vi "v5.41.vi"() -> ()   [LabVIEW 2018]
uses:
  <vilib>/DAQmx/read.llb/DAQmx Read (Analog 1D DBL NChan 1Samp).vi
  <extravilib>/ChannelInstances/Lossy Stream-c(a[.](c(dbl,dbl,dbl,dbl)),stamp,a[.](dbl),c(dbl,dbl,dbl,dbl,dbl,dbl,dbl))/Read With Abort.vi
  <extravilib>/ChannelInstances/High Speed Stream-c(a[.](c(dbl,dbl,dbl,dbl)),stamp,a[.](dbl),c(dbl,dbl,dbl,dbl,dbl,dbl,dbl))/_Read For Replicate.vi
  <extravilib>/ChannelInstances/Lossy Stream-c(a[.](c(dbl,dbl,dbl,dbl)),stamp,a[.](dbl),c(dbl,dbl,dbl,dbl,dbl,dbl,dbl))/Write With Abort.vi
  <extravilib>/ChannelInstances/Lossy Stream-c(a[.](c(dbl,dbl,dbl,dbl)),stamp,a[.](dbl),c(dbl,dbl,dbl,dbl,dbl,dbl,dbl))/EndpointRead.vi
  <extravilib>/ChannelInstances/Lossy Stream-c(a[.](c(dbl,dbl,dbl,dbl)),stamp,a[.](dbl),c(dbl,dbl,dbl,dbl,dbl,dbl,dbl))/Endpoint.vi
  <extravilib>/ChannelInstances/Lossy Stream-c(a[.](c(dbl,dbl,dbl,dbl)),stamp,a[.](dbl),c(dbl,dbl,dbl,dbl,dbl,dbl,dbl))/Instantiate.vi
  <extravilib>/ChannelInstances/Lossy Stream-c(a[.](c(dbl,dbl,dbl,dbl)),stamp,a[.](dbl),c(dbl,dbl,dbl,dbl,dbl,dbl,dbl))/)Channel.vi
  <resource>/ChannelSupport/_ChannelSupport/WaitIfNeeded.vi
  <extravilib>/ChannelInstances/High Speed Stream-c(a[.](c(dbl,dbl,dbl,dbl)),stamp,a[.](dbl),c(dbl,dbl,dbl,dbl,dbl,dbl,dbl))/Instantiate.vi
  <extravilib>/ChannelInstances/High Speed Stream-c(a[.](c(dbl,dbl,dbl,dbl)),stamp,a[.](dbl),c(dbl,dbl,dbl,dbl,dbl,dbl,dbl))/)Channel.vi
  <extravilib>/ChannelInstances/High Speed Stream-c(a[.](c(dbl,dbl,dbl,dbl)),stamp,a[.](dbl),c(dbl,dbl,dbl,dbl,dbl,dbl,dbl))/Abort Signal/Init Signal.vi
  <vilib>/Utility/file.llb/Write Delimited Spreadsheet (string).vi
  <vilib>/DAQmx/create/channels.llb/DAQmx Create Channel (AI-Temperature-Thermocouple).vi
  <vilib>/DAQmx/configure/timing.llb/DAQmx Timing (Sample Clock).vi
  <vilib>/DAQmx/miscellaneous.llb/DAQmx Fill In Error Info.vi
  <extravilib>/ChannelInstances/High Speed Stream-c(a[.](c(dbl,dbl,dbl,dbl)),stamp,a[.](dbl),c(dbl,dbl,dbl,dbl,dbl,dbl,dbl)).lvlib
  <resource>/objmgr/daqmx.rc
  <extravilib>/ChannelInstances/Lossy Stream-c(a[.](c(dbl,dbl,dbl,dbl)),stamp,a[.](dbl),c(dbl,dbl,dbl,dbl,dbl,dbl,dbl)).lvlib
panel:
  in  "Rig Temperature Tab Box":enum32{"Rig Temps Live", "Alarm Thresholds"}(tab)
  out "Rig Temperatures":T1
  in  "Rig Alarm Thresholds":T1
  out "DAQ Current Time":timestamp format="%<%X>T"
  in  "UI Refresh Rate (Hz)":u32=1 min=1 max=500 step=1
  out "Line Pressures":T2(graph)
  in  "Boondoggle":dbl(slide) scale=0.0..10.0
  out "Line Temperatures":T2(graph)
  out "Stoichiometric AFR [g/s]":dbl
  in  "stop":bool
  in  "Species List":string[][](table)=[["Custom", "9999999999"], ["Methanol", "6.47"], ["Butanol", "11.2"], ["Diesel", "14.5"], ["Gasoline", "14.7"], ["Propane", "15.67"], ["Methane", "13.19"], ["Hydrogen", "34.3"], ["Ammonia", "6.0466"], ["Pentane", "15.32"], ["Butane", "14.98"], ["Hexane", "15.24"], ["Ethanol", "9"], ["Empty (Not Used)", "0"]]
  in  "Lines Tab Control\n(Don't delete)":enum32{"Live Data", "AFR Info", "Setup Lines"}(tab)
  out "Flowrate Data":T3(array[cluster])
  out "AFR Display":T4(array[cluster])
  in  "Line Setup":T5(array[cluster])
  out "Actual Sample Rate":dbl
  out "Export Timestamp":timestamp format="%<%H:%M:%S>T"
  out "UI Timestamp":timestamp format="%<%X\n%x>T"
  in  "file path (dialog if empty)":path
  out "Export Loop Status":T6(ring)
  in  "Start Recording?":bool
  in  "Stop Recording?":bool
  out "Aquisition\nLoop Status":T7(ring)
  in  "OK Button":bool
  in  "DAQ Properties":cluster{"Sample Rate [Hz]":dbl}={"Sample Rate [Hz]"=1.0} {"Sample Rate [Hz]" min=1.0 max=500.0 step=1.0}
  # "Rig Temperatures [ °C]"
  # "Rig Alarm Thresholds [ °C]"
  # "Live \n Live Line Data"
  # "Air-to-Fuel Ratios for each Line"
  # "Line Setup"
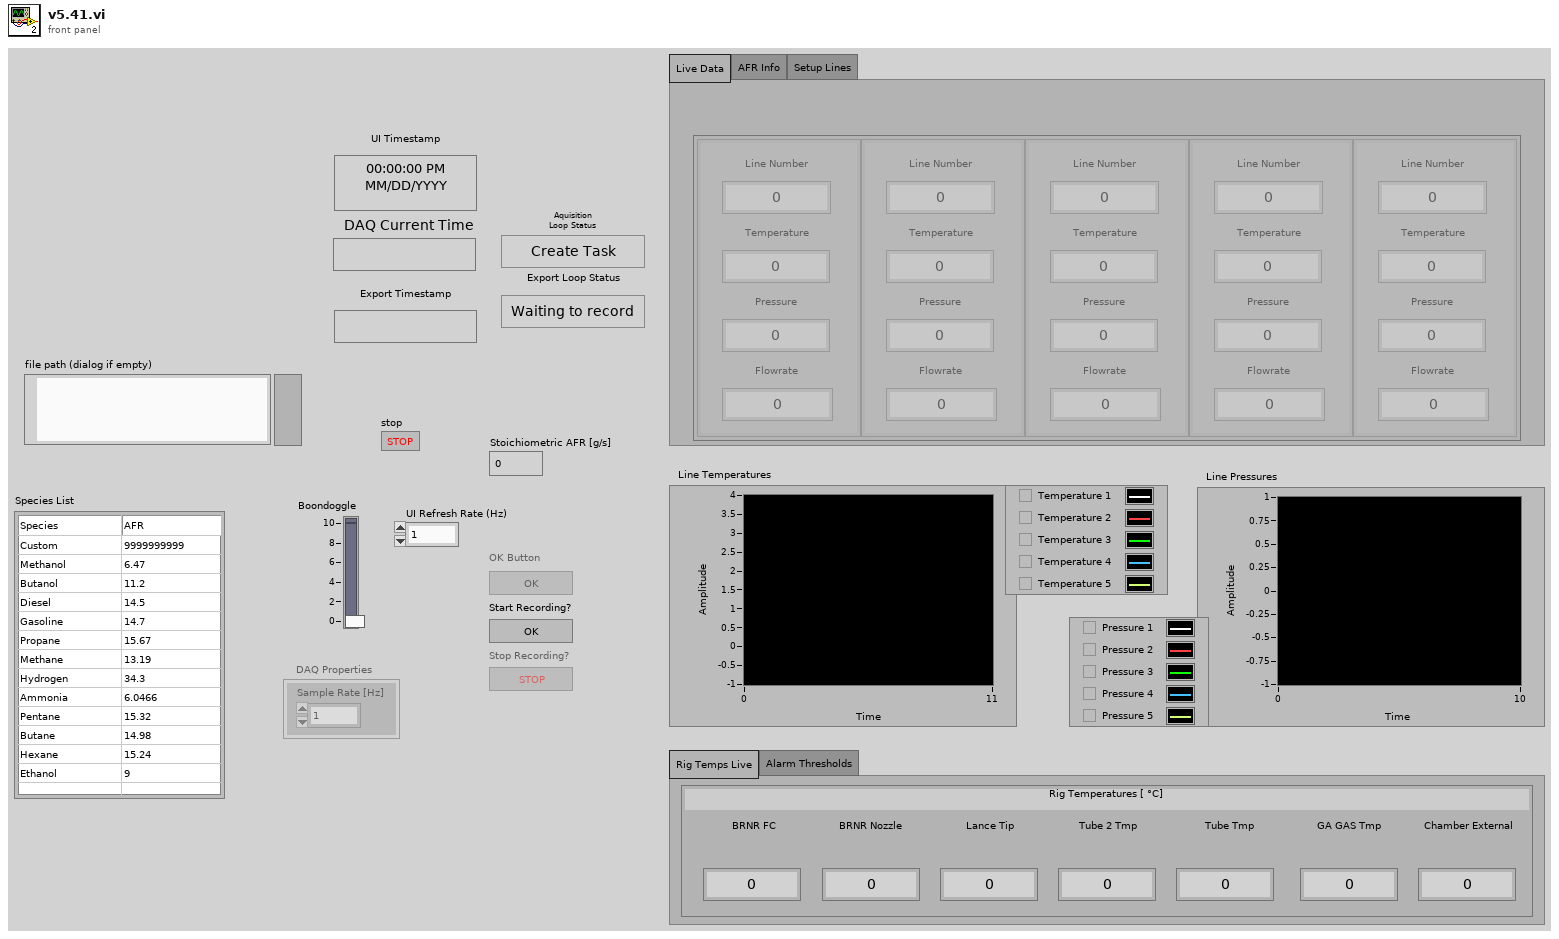
[diagram p1: front panel]
types:
  T1 = cluster{"BRNR FC":dbl, "BRNR Nozzle":dbl, "Lance Tip":dbl, "Tube 2 Tmp":dbl, "Tube Tmp":dbl, "GA GAS Tmp":dbl, "Chamber External":dbl}
  T2 = cluster{"[0]":dbl, "[1]":dbl, "[2]":dbl, "[3]":dbl, "[4]":dbl}
  T3 = cluster{"Line Number":dbl, "Temperature":dbl, "Pressure":dbl, "Flowrate":dbl}[]
  T4 = cluster{"Line Number":i32, "AFR":dbl, "Species":enum16{"Empty (Not used)", "Custom", "Methanol", "Ethanol", "Butanol", "Diesel", "Gasoline", "Propane", "Methane", "Hydrogen", "Pentane", "Butane", "Hexane"}}[]
  T5 = cluster{"Custom AFR":dbl, "Species":enum16{"Empty (Not used)", "Custom", "Methanol", "Ethanol", "Butanol", "Diesel", "Gasoline", "Propane", "Methane", "Hydrogen", "Pentane", "Butane", "Hexane"}}[]
  T6 = enum16{"Waiting to record", "Creating Spreadsheet", "Recording", "Finished Recording"}
  T7 = enum16{"Create Task", "Change Settings", "Check Settings", "Read Data", "End Task"}
  T8 = enum8{"Enabled", "Disabled", "Disabled and Grayed Out"}
  T9 = cluster{"Line":i32, "AFR":dbl, "Species":enum16{"Empty (Not used)", "Custom", "Methanol", "Ethanol", "Butanol", "Diesel", "Gasoline", "Propane", "Methane", "Hydrogen", "Pentane", "Butane", "Hexane"}}
  T10 = enum16{"Empty (Not used)", "Custom", "Methanol", "Ethanol", "Butanol", "Diesel", "Gasoline", "Propane", "Methane", "Hydrogen", "Pentane", "Butane", "Hexane"}
  T11 = cluster{"Flowrate Data":cluster{"Line Number":dbl, "Temperature":dbl, "Pressure":dbl, "Flowrate":dbl}[], "Current Time":timestamp, "DAQmx Data":dbl[], "Rig Temperatures":cluster{"BRNR FC":dbl, "BRNR Nozzle":dbl, "Lance Tip":dbl, "Tube 2 Tmp":dbl, "Tube Tmp":dbl, "GA GAS Tmp":dbl, "Chamber External Temp":dbl}}
  T12 = cluster{"BRNR FC":dbl, "BRNR Nozzle":dbl, "Lance Tip":dbl, "Tube 2 Tmp":dbl, "Tube Tmp":dbl, "GA GAS Tmp":dbl, "Chamber External Temp":dbl}
  T13 = typedef "High Speed Stream-c(a[.](c(dbl,dbl,dbl,dbl)),stamp,a[.](dbl),c(dbl,dbl,dbl,dbl,dbl,dbl,dbl)).lvlib/)Channel.ctl" = refnum<queue>
  T14 = typedef "Lossy Stream-c(a[.](c(dbl,dbl,dbl,dbl)),stamp,a[.](dbl),c(dbl,dbl,dbl,dbl,dbl,dbl,dbl)).lvlib/)Channel.ctl" = refnum<queue>
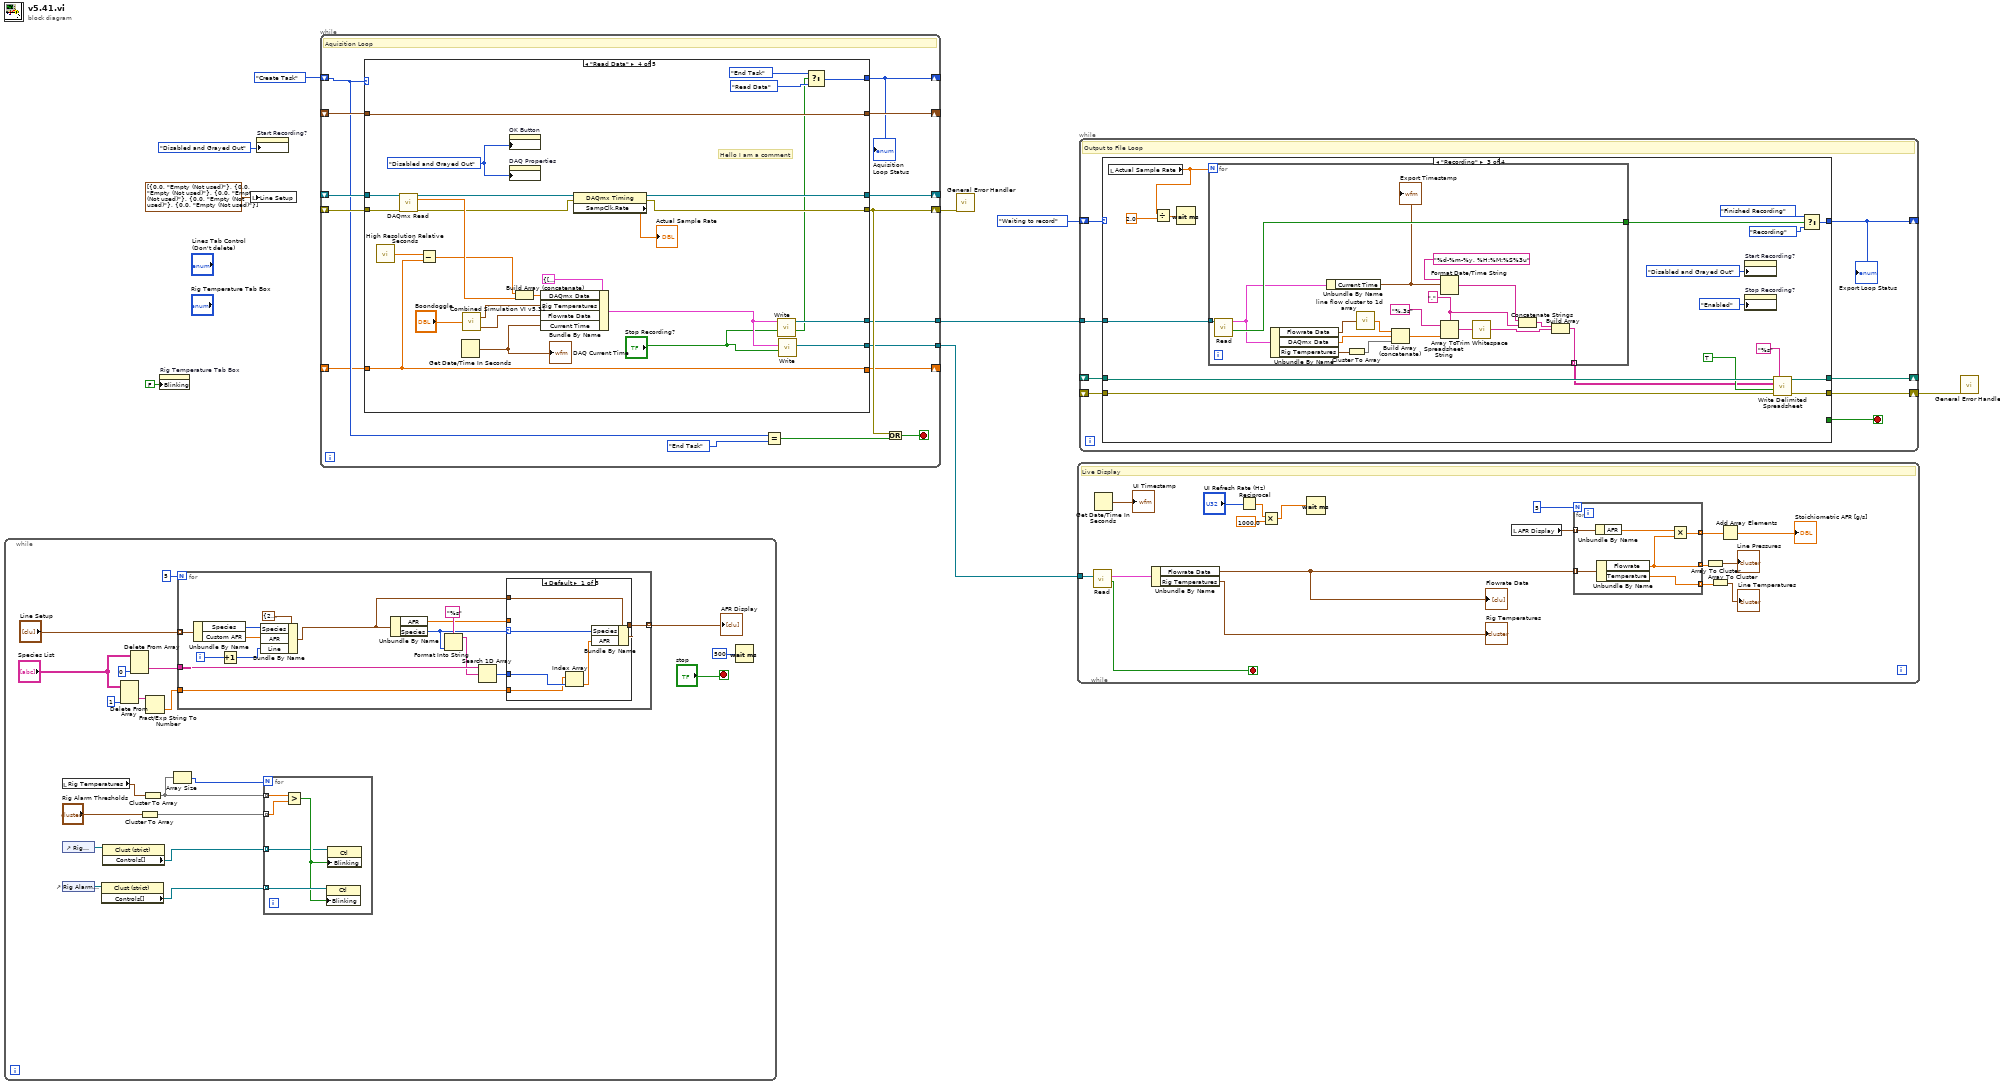
[diagram p0: block diagram]
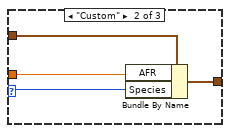
[diagram p2: hidden frame]
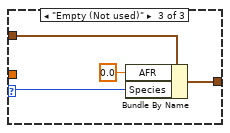
[diagram p3: hidden frame]
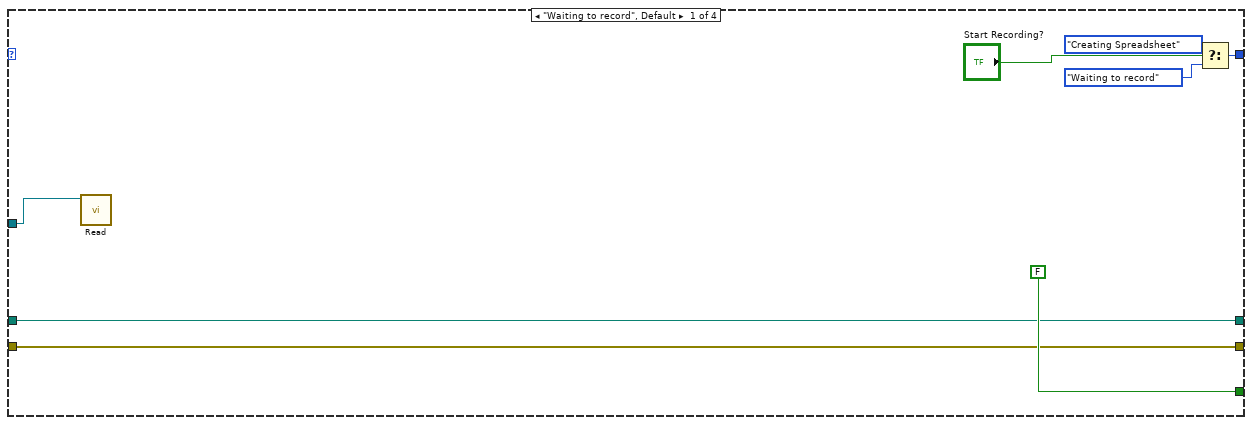
[diagram p4: hidden frame]
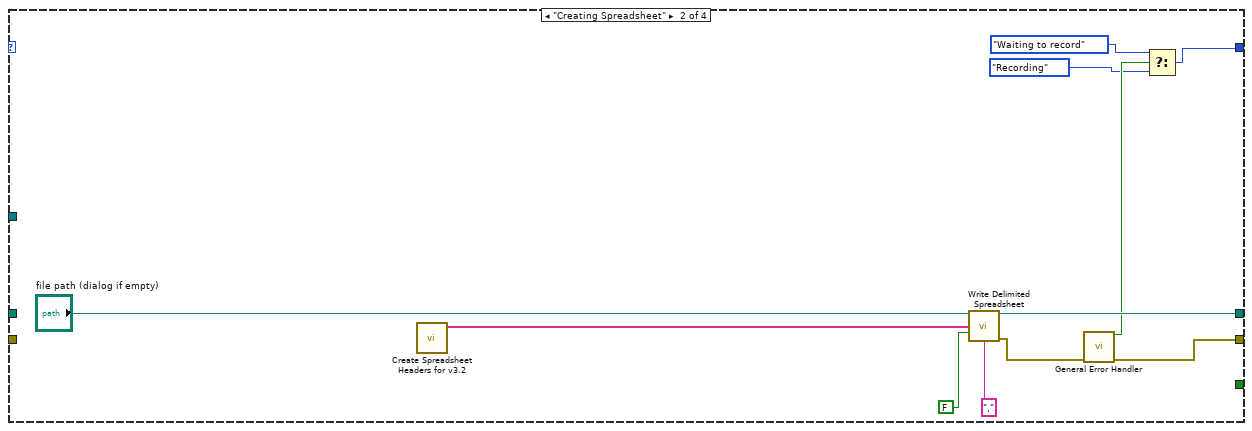
[diagram p5: hidden frame]
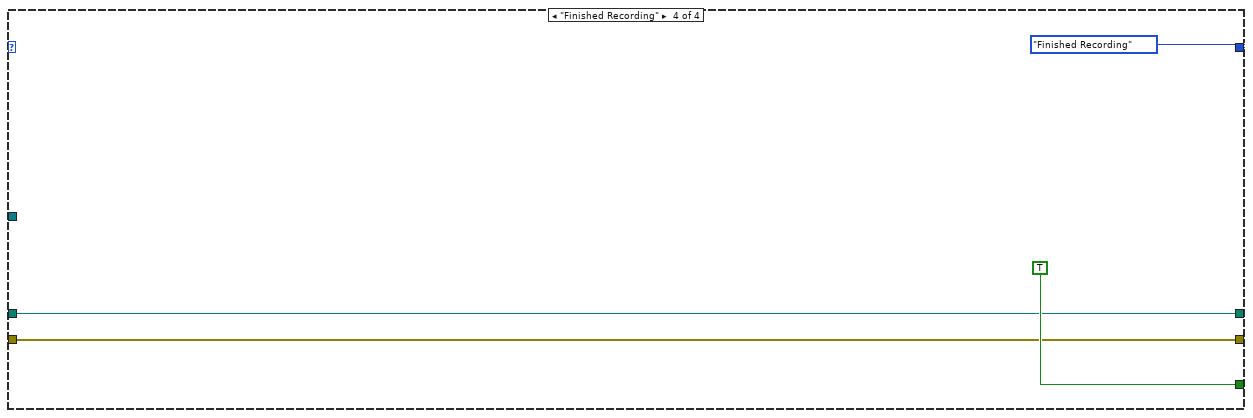
[diagram p6: hidden frame]
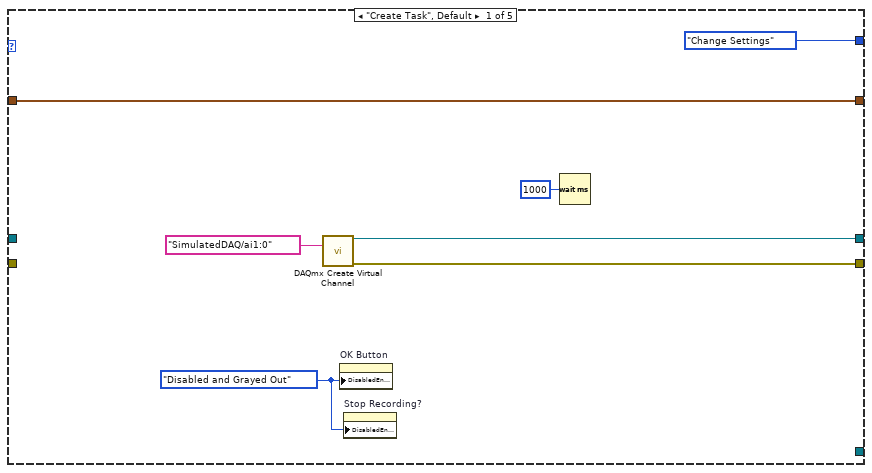
[diagram p7: hidden frame]
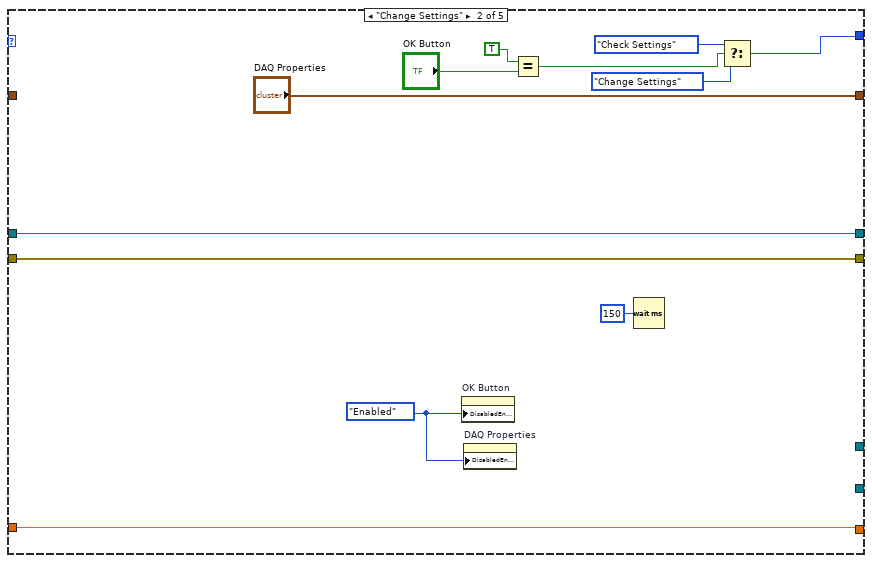
[diagram p8: hidden frame]
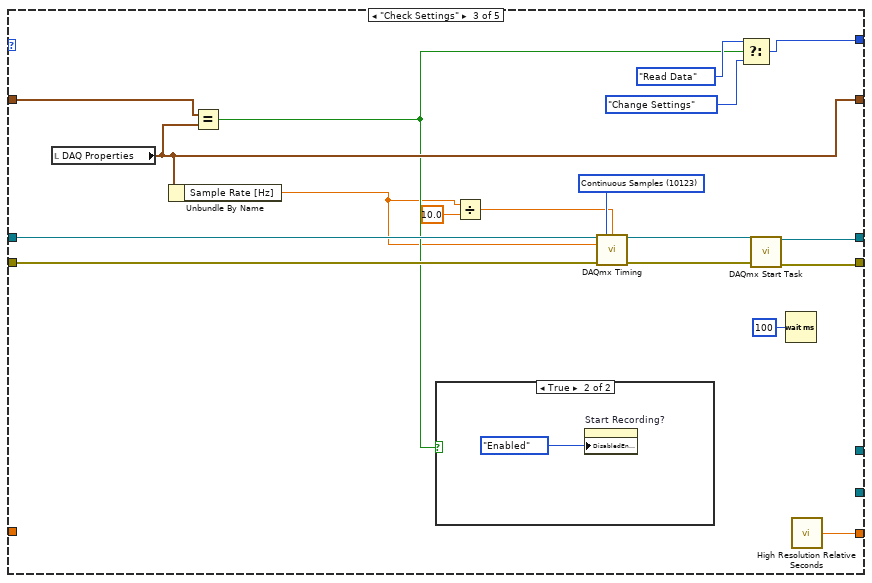
[diagram p9: hidden frame]
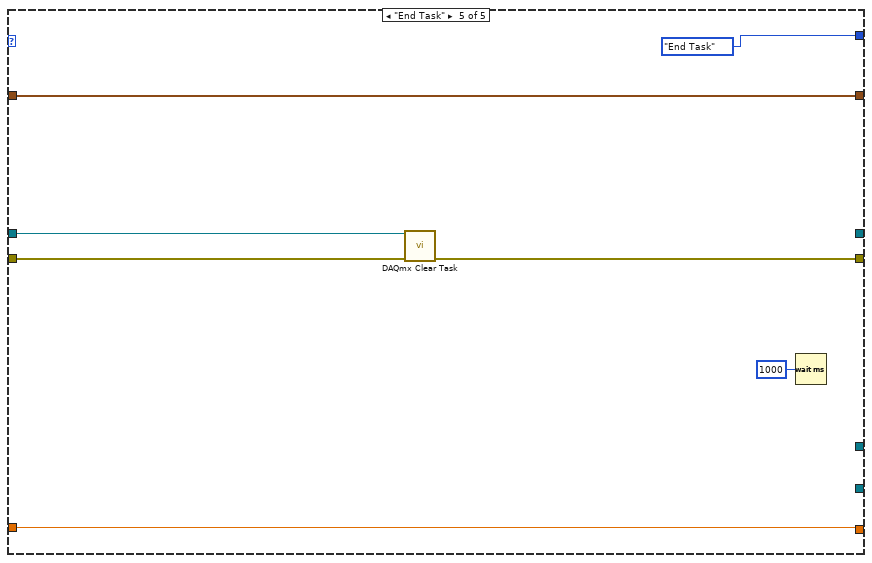
[diagram p11: hidden frame]
diagram:
  n1 = while {
    stop <- "stop" stop-if-true
    n2 = local read "Rig Temperatures"() -> (w17:T1)
    n3 = control-ref of="Rig Temperatures"() -> (w13:refnum<vi>)
    n4 = control-ref of="Rig Alarm Thresholds"() -> (w12:refnum<vi>)
    n5 = property class="Clust (strict)"(reference=w12) -> ("Controls[]"=w11:refnum<vi>[])  [unwired: 1 in, 2 out]
    n6 = property class="Clust (strict)"(reference=w13) -> ("Controls[]"=w10:refnum<vi>[])  [unwired: 1 in, 2 out]
    n7 = Delete From Array(array="Species List", index (col)=1 ("disabled index (col)")) -> (deleted portion=w24:string[])  [unwired: 2 in, 1 out]
    n8 = Delete From Array(array="Species List", index (col)=0) -> (deleted portion=w25:string[])  [unwired: 2 in, 1 out]
    n9 = Cluster To Array(cluster="Rig Alarm Thresholds") -> (array=w16:dbl[])
    n10 = Cluster To Array(cluster=w17) -> (array=w14:dbl[])
    n11 = Fract/Exp String To Number(string=w24) -> (number=w23:dbl[])  [unwired: 3 in, 1 out]
    n12 = Array Size(array=w14) -> (size(s)=w15:i32)
    n13 = for {
      N: 5 -> [_]
      tunnel: w25 -> [w48]
      tunnel: w23 -> [w45]
      tunnel: "Line Setup" -> [w38] mode=indexing
      tunnel: [w35] -> w19 mode=indexing
      i -> [w37]
      n14 = Unbundle By Name(w38) -> ("Species"=w42:T10, "Custom AFR"=w41:dbl)
      n15 = Increment(x=w37) -> (x+1=w39:i32)
      n16 = Bundle By Name(cluster=T9 {"Line"=2, "AFR"=1.0, "Species"=enum."Pentane"} ("AFR Inputs"), "Species"=w42, "AFR"=w41, "Line"=w39) -> (w36:T9)
      n17 = Unbundle By Name(w36) -> ("AFR"=w46:dbl, "Species"=w43:T10)
      n18 = Format Into String(format string="%s", w43) -> (resulting string=w47:string)  [unwired: 2 in, 1 out]
      n19 = Search 1D Array(1D array=w48, element=w47) -> (index of element=w44:i32)  [unwired: 1 in]
      n20 = case shown="Default" w43 {
        selector: w43 -> [w52 w56 w61]
        tunnel: w46 -> [_ w59 _]
        tunnel: w45 -> [w54 _ _]
        tunnel: w44 -> [w55 _ _]
        tunnel: [w50 w58 w63] -> w35
        tunnel: w36 -> [w51 w57 w62]
        frame Default {
          n21 = Index Array(array=w54, index=w55) -> (element=w53:dbl)
          n22 = Bundle By Name(cluster=w51, "Species"=w52, "AFR"=w53) -> (w50:T9)
        }
        frame "Custom" {
          n23 = Bundle By Name(cluster=w57, "AFR"=w59, "Species"=w56) -> (w58:T9)
        }
        frame "Empty (Not used)" {
          n24 = Bundle By Name(cluster=w62, "AFR"=0.0, "Species"=w61) -> (w63:T9)
        }
      }
    }
    "AFR Display" <- w19
    n25 = for {
      N: w15 -> [_]
      tunnel: w16 -> [w33] mode=indexing
      tunnel: w14 -> [w34] mode=indexing
      tunnel: w11 -> [w32] mode=indexing
      tunnel: w10 -> [w30] mode=indexing
      n26 = Greater?(x=w34, y=w33) -> (0:w31:bool)
      n27 = property on="Property Node" class="Ctl"(reference=w32, "Blinking"=w31) -> ()  [unwired: 1 in, 2 out]
      n28 = property on="Property Node" class="Ctl"(reference=w30, "Blinking"=w31) -> ()  [unwired: 1 in, 2 out]
    }
    n29 = Wait (ms)(milliseconds to wait=u32 500) -> ()  [unwired: 1 out]
  }
  n30 = property on="Rig Temperature Tab Box" class="TabCtl (strict)"("Blinking"=FALSE) -> ()  [unwired: 2 in, 2 out]
  n31 = local write "Line Setup"(T5 [{"Custom AFR"=0.0, "Species"=enum."Empty (Not used)"}, {"Custom AFR"=0.0, "Species"=enum."Empty (Not used)"}, {"Custom AFR"=0.0, "Species"=enum."Empty (Not used)"}, {"Custom AFR"=0.0, "Species"=enum."Empty (Not used)"}, {"Custom AFR"=0.0, "Species"=enum."Empty (Not used)"}] ("Line Setup 2")) -> ()
  n32 = property on="Start Recording?" class="Bool"("DisabledEnum"=T8."Disabled and Grayed Out" ("Disabled")) -> ()  [unwired: 2 in, 2 out]
  n33 = while {
    shift-right: [w73] -> _
    shift-left: T7."Create Task" -> [w69]
    shift-right: [w78] -> _
    shift-left: _ -> [w76]
    shift-right: [w72] -> w5
    shift-left: _ -> [w75]
    shift-right: [w77] -> _
    shift-left: _ -> [w74]
    tunnel: [w68] -> w7
    tunnel: [w66] -> w3
    shift-right: [w64] -> _
    shift-left: _ -> [w65]
    stop <- w67 stop-if-true
    # "Aquisition Loop"
    n34 = case shown="\"Read Data\"" w69 {
      tunnel: [w85 w97 w105 w130 _] -> w78
      tunnel: [w84 w96 w104 w131 w150] -> w72
      tunnel: [T7."Change Settings" w90 w111 w139 T7."End Task"] -> w73
      tunnel: [w81 "DAQ Properties" w108 w141 w149] -> w77
      tunnel: w76 -> [_ w97 w110 w143 w147]
      tunnel: w75 -> [_ w96 w109 w142 w146]
      tunnel: w74 -> [w81 _ w115 w141 w149]
      tunnel: [_ _ _ w135 _] -> w68
      tunnel: [_ w86 w98 w126 w144] -> w64
      tunnel: w65 -> [_ w86 _ w126 w144]
      tunnel: [_ _ _ w123 _] -> w66
      frame "Create Task", Default {
        w79 = T8."Disabled and Grayed Out" ("Disabled")
        n35 = call-poly <vilib>:"DAQmx Create Virtual Channel.vi"("physical channels"=tag "SimulatedDAQ/ai1:0") -> ("task out"=w85:refnum<k21>, "error out"=w84:errorcluster)  [unwired: 13 in]
        n36 = property on="OK Button" class="Bool"("DisabledEnum"=w79) -> ()  [unwired: 2 in, 2 out]
        n37 = property on="Stop Recording?" class="Bool"("DisabledEnum"=w79) -> ()  [unwired: 2 in, 2 out]
        n38 = Wait (ms)(milliseconds to wait=u32 1000) -> ()  [unwired: 1 out]
      }
      frame "Change Settings" {
        w87 = T8."Enabled" ("Disabled")
        n39 = property on="OK Button" class="Bool"("DisabledEnum"=w87) -> ()  [unwired: 2 in, 2 out]
        n40 = property on="DAQ Properties" class="Clust (strict)"("DisabledEnum"=w87) -> ()  [unwired: 2 in, 2 out]
        n41 = Equal?(x=TRUE, y="OK Button") -> (x = y?=w92:bool)
        n42 = Wait (ms)(milliseconds to wait=u32 150) -> ()  [unwired: 1 out]
        n43 = Select(t=T7."Check Settings", s=w92, f=T7."Change Settings") -> (s? t:f=w90:T7)
      }
      frame "Check Settings" {
        w103 = 10123 items=["Finite Samples"=10178, "Continuous Samples"=10123, "Hardware Timed Single Point"=12522] ("sample mode")
        n44 = local read "DAQ Properties"() -> (w108:cluster{"Sample Rate [Hz]":dbl})
        n45 = Unbundle By Name(w108) -> ("Sample Rate [Hz]"=w100:dbl)
        n46 = Equal?(x=w115, y=w108) -> (x = y?=w102:bool)
        n47 = case shown="True" w102 {
          frame False {
          }
          frame True {
            n48 = property on="Start Recording?" class="Bool"("DisabledEnum"=T8."Enabled" ("Disabled")) -> ()  [unwired: 2 in, 2 out]
          }
        }
        n49 = Divide(x=w100, y=10.0) -> (x/y=w99:dbl)
        n50 = call-poly <vilib>:"DAQmx Timing.vi"("task/channels in"=w110, "sample mode"=w103, "samples per channel"=w99, "rate"=w100, "error in"=w109) -> ("task out"=w107:refnum<k21>, "error out"=w106:errorcluster)  [unwired: 9 in]
        n51 = Select(t=T7."Read Data", s=w102, f=T7."Change Settings") -> (s? t:f=w111:T7)
        n52 = call <vilib>:"DAQmx Start Task.vi"("task/channels in"=w107, "error in"=w106) -> ("task out"=w105:refnum<k21>, "error out"=w104:errorcluster)  [unwired: 12 in]
        n53 = Wait (ms)(milliseconds to wait=u32 100) -> ()  [unwired: 1 out]
        n54 = call <vilib>:"High Resolution Relative Seconds.vi"() -> ("relative seconds"=w98:dbl)
      }
      frame "Read Data" {
        w134 = T8."Disabled and Grayed Out" ("Disabled")
        # "Hello I am a comment"
        n55 = call <vilib>:"High Resolution Relative Seconds.vi"() -> ("relative seconds"=w128:dbl)
        n56 = call-poly <vilib>:"DAQmx Read.vi"("task/channels in"=w143, "error in"=w142) -> ("task out"=w132:refnum<k21>, "data"=w137:dbl[], "error out"=w129:errorcluster)  [unwired: 11 in]
        n57 = Subtract(x=w128, y=w126) -> (x-y=w127:dbl)
        n58 = Get Date/Time In Seconds() -> (seconds since 1Jan1904=w118:timestamp)
        "DAQ Current Time" <- w118
        n59 = call "Combined Simulation VI v5.31.vi"("Boondoggle Input"="Boondoggle") -> ("Rig Temperatures Cluster"=w117:T12, "Line Data (Array of Clusters)"=w119:T3)
        n60 = property on="OK Button" class="Bool"("DisabledEnum"=w134) -> ()  [unwired: 2 in, 2 out]
        n61 = property on="DAQ Properties" class="Clust (strict)"("DisabledEnum"=w134) -> ()  [unwired: 2 in, 2 out]
        n62 = Build Array (concatenate)(w127, w137) -> (w121:dbl[])
        n63 = Bundle By Name(cluster=T11 {"Flowrate Data"=[{"Line Number"=1.0, "Temperature"=17.480721541683437, "Pressure"=24.0, "Flowrate"=0.0}, {"Line Number"=2.0, "Temperature"=21.850901927104296, "Pressure"=30.0, "Flowrate"=0.0}, {"Line Number"=3.0, "Temperature"=26.221082312525155, "Pressure"=36.0, "Flowrate"=0.0}, {"Line Number"=4.0, "Temperature"=30.591262697946018, "Pressure"=42.00000000000001, "Flowrate"=0.0}, {"Line Number"=5.0, "Temperature"=34.96144308336687, "Pressure"=48.0, "Flowrate"=0.0}], "Current Time"=timestamp(0 s since 1904-01-01), "DAQmx Data"=[], "Rig Temperatures"={"BRNR FC"=0.0, "BRNR Nozzle"=0.0, "Lance Tip"=0.0, "Tube 2 Tmp"=0.0, "Tube Tmp"=0.0, "GA GAS Tmp"=0.0, "Chamber External Temp"=0.0}}, "DAQmx Data"=w121, "Rig Temperatures"=w117, "Flowrate Data"=w119, "Current Time"=w118) -> (w133:T11)
        n64 = property class="DAQmx Timing"(reference=w132, error in=w129) -> (reference out=w130:refnum<k21>, error out=w131:errorcluster, "SampClk.Rate"=→"Actual Sample Rate":dbl)
        n65 = call <extravilib>:"Write.vi"("last element? (F)"="Stop Recording?", "element"=w133) -> ("done?"=w122:bool, "channel"=w135:T13)  [unwired: 7 in, 1 out]
        n66 = call <extravilib>:"Write.vi"("last element? (F)"="Stop Recording?", "element"=w133) -> ("channel"=w123:T14)  [unwired: 7 in, 2 out]
        n67 = Select(t=T7."End Task", s=w122, f=T7."Read Data") -> (s? t:f=w139:T7)
      }
      frame "End Task" {
        n68 = call <vilib>:"DAQmx Clear Task.vi"("task in"=w147, "error in"=w146) -> ("error out"=w150:errorcluster)  [unwired: 13 in]
        n69 = Wait (ms)(milliseconds to wait=u32 1000) -> ()  [unwired: 1 out]
      }
    }
    "Aquisition\nLoop Status" <- w73
    n70 = Equal?(x=w69, y=T7."End Task") -> (x = y?=w70:bool)
    n71 = Or(x=w72, y=w70) -> (x .or. y?=w67:bool)
  }
  n72 = call <vilib>:"General Error Handler.vi"("error in (no error)"=w5) -> ()  [unwired: 10 in, 5 out]
  n73 = while {
    tunnel: w3 -> [w159]
    stop <- w155 stop-if-true
    # "Live Display"
    n74 = call <extravilib>:"Read.vi"("channel"=w159) -> ("last element?"=w155:bool, "element"=w158:T11)  [unwired: 5 in, 4 out]
    n75 = Get Date/Time In Seconds() -> (seconds since 1Jan1904=→"UI Timestamp":timestamp)
    n76 = Unbundle By Name(w158) -> ("Flowrate Data"=w156:T3, "Rig Temperatures"=→"Rig Temperatures":T12)
    "Flowrate Data" <- w156
    n77 = Reciprocal(x="UI Refresh Rate (Hz)") -> (1/x=w152:dbl)
    n78 = Multiply(x=w152, y=1000.0) -> (x*y=w151:dbl)
    n79 = Wait (ms)(milliseconds to wait=w151) -> ()  [unwired: 1 out]
    n80 = local read "AFR Display"() -> (w166:T4)
    n81 = for {
      N: 5 -> [_]
      tunnel: w166 -> [w174] mode=indexing
      tunnel: [w172] -> w165 mode=indexing
      tunnel: [w171] -> w162 mode=indexing
      tunnel: [w170] -> w163 mode=indexing
      tunnel: w156 -> [w169] mode=indexing
      n82 = Unbundle By Name(w174) -> ("AFR"=w173:dbl)
      n83 = Unbundle By Name(w169) -> ("Flowrate"=w170:dbl, "Temperature"=w171:dbl)
      n84 = Multiply(x=w173, y=w170) -> (x*y=w172:dbl)
    }
    n85 = Array To Cluster(array=w163) -> (cluster=→"Line Pressures":T2)
    n86 = Array To Cluster(array=w162) -> (cluster=→"Line Temperatures":T2)
    n87 = Add Array Elements(numeric array=w165) -> (sum=→"Stoichiometric AFR [g/s]":dbl)
  }
  n88 = while {
    shift-right: [w182] -> _
    shift-left: T6."Waiting to record" -> [w181]
    tunnel: w7 -> [w179]
    shift-right: [w177] -> _
    shift-left: _ -> [w178]
    shift-right: [w176] -> w6
    shift-left: _ -> [w175]
    stop <- w180 stop-if-true
    # "Output to File Loop"
    n89 = case shown="\"Recording\"" w181 {
      tunnel: [w187 w193 w217 T6."Finished Recording"] -> w182
      tunnel: [FALSE _ _ TRUE] -> w180
      tunnel: w179 -> [w183 _ w214 _]
      tunnel: w178 -> [w185 _ w211 w238]
      tunnel: [w185 w201 w212 w238] -> w177
      tunnel: [w184 w195 w207 w237] -> w176
      tunnel: w175 -> [w184 _ w210 w237]
      frame "Waiting to record", Default {
        n90 = call <extravilib>:"Read.vi"("channel"=w183) -> ()  [unwired: 6 in, 5 out]
        n91 = Select(t=T6."Creating Spreadsheet", s="Start Recording?", f=T6."Waiting to record") -> (s? t:f=w187:T6)
      }
      frame "Creating Spreadsheet" {
        n92 = call "Create Spreadsheet Headers for v3.2.vi"() -> ("Array"=w200:string[])  [unwired: 11 in]
        n93 = call-poly <vilib>:"Write Delimited Spreadsheet.vi"("file path (dialog if empty)"="file path (dialog if empty)", "1D data"=w200, "append to file? (new file:F)"=FALSE, "delimiter (\\t)"="," ("delimiter (\\t)")) -> ("new file path (Not A Path if cancelled)"=w201:path, "error out"=w196:errorcluster)  [unwired: 10 in]
        n94 = call <vilib>:"General Error Handler.vi"("error in (no error)"=w196) -> ("error?"=w194:bool, "error out"=w195:errorcluster)  [unwired: 10 in, 3 out]
        n95 = Select(t=T6."Waiting to record", s=w194, f=T6."Recording") -> (s? t:f=w193:T6)
      }
      frame "Recording" {
        n96 = local read "Actual Sample Rate"() -> (w203:dbl)
        n97 = Divide(x=w203, y=2.0) -> (x/y=w202:dbl)
        n98 = Wait (ms)(milliseconds to wait=w202) -> ()  [unwired: 1 out]
        n99 = for {
          N: w203 -> [_]
          tunnel: w214 -> [w235]
          tunnel: [w234] -> w213
          tunnel: [w219] -> w205 mode=indexing
          w224 = "," ("delimiter (Tab)")
          n100 = call <extravilib>:"Read.vi"("channel"=w235) -> ("done?"=w234:bool, "element"=w232:T11)  [unwired: 6 in, 3 out]
          n101 = Unbundle By Name(w232) -> ("Flowrate Data"=w233:T3, "DAQmx Data"=w230:dbl[], "Rig Temperatures"=w236:T12)
          n102 = Unbundle By Name(w232) -> ("Current Time"=w225:timestamp)
          "Export Timestamp" <- w225
          n103 = Cluster To Array(cluster=w236) -> (array=w231:dbl[])
          n104 = call "line flow cluster to 1d array.vi"("Flowrate Data"=w233) -> ("Array"=w229:dbl[])
          n105 = Build Array (concatenate)(w229, w230, w231) -> (w222:dbl[])
          n106 = Format Date/Time String(time format string (%c)="%d-%m-%y, %H:%M:%S%3u", seconds (now)=w225) -> (date/time string=w223:string)  [unwired: 1 in]
          n107 = Array To Spreadsheet String(delimiter (Tab)=w224, array=w222, 3:"%.3s" ("format string")) -> (spreadsheet string=w228:string)
          n108 = call <vilib>:"Trim Whitespace.vi"("string"=w228) -> ("trimmed string"=w220:string)  [unwired: 1 in]
          n109 = Concatenate Strings(w223, w224) -> (w221:string)
          n110 = Build Array(w221, w220) -> (w219:string[])
        }
        n111 = property on="Start Recording?" class="Bool"("DisabledEnum"=T8."Disabled and Grayed Out" ("Disabled")) -> ()  [unwired: 2 in, 2 out]
        n112 = property on="Stop Recording?" class="Bool"("DisabledEnum"=T8."Enabled" ("Disabled")) -> ()  [unwired: 2 in, 2 out]
        n113 = call-poly <vilib>:"Write Delimited Spreadsheet.vi"("file path (dialog if empty)"=w211, "format (%s)"="%s", "2D data"=w205, "append to file? (new file:F)"=TRUE, "error in (no error)"=w210) -> ("new file path (Not A Path if cancelled)"=w212:path, "error out"=w207:errorcluster)  [unwired: 9 in]
        n114 = Select(t=T6."Finished Recording", s=w213, f=T6."Recording") -> (s? t:f=w217:T6)
      }
      frame "Finished Recording" {
      }
    }
    "Export Loop Status" <- w182
  }
  n115 = call <vilib>:"General Error Handler.vi"("error in (no error)"=w6) -> ()  [unwired: 10 in, 5 out]
